vi "FTW-CodeGen-GenerateCode.vi"(0 "State In":T2, 5 "XRef":refnum<vi>, 7 "Terms":T1(array[cluster]), 9 "Diagram":refnum<vi>) -> (4 "State Out":T2, 6 "Reply":string[](array[string]), 8 "Generated Code?":bool)   [LabVIEW 2013, in "FTW-SQLite-Insert.xnode"]
uses:
  FTW-SQLite-Insert.xnode
  FTW-CodeGen-State.ctl
  codegen/FTW-CodeGen.lvlib
panel:
  # "Inputs"
  # "Outputs"
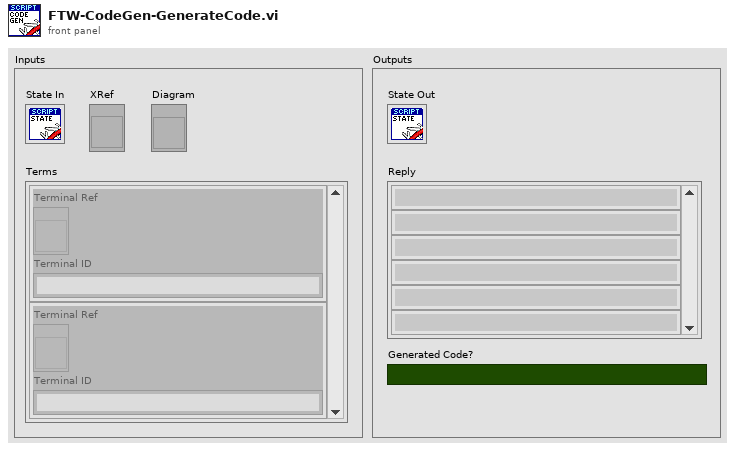
[diagram p1: front panel]
types:
  T1 = cluster{"Terminal Ref":refnum<vi>, "Terminal ID":string}[]
  T2 = typedef "FTW-SQLite-Insert.xnode/FTW-CodeGen-State.ctl" = cluster{"Dummy":string}
  T3 = typedef "LVPositionTypeDef.ctl" = cluster{"Left":i32, "Top":i32}
  T4 = typedef "FTW-Reflection-Types.ctl" = enum16{"Unknown", "Void", "Array", "Cluster", "LVObject", "Boolean", "I8", "I16", "I32", "I64", "U8", "U16", "U32", "U64", "SGL", "DBL", "EXT", "CSG", "CDB", "CXT", "FXP", "EnumU8", "EnumU16", "EnumU32", "EnumU64", "SGLwithUnit", "DBLwithUnit", "EXTwithUnit", "CSGwithUnit", "CDBwithUnit", "CXTwithUnit", "String", "Path", "Picture", "Tag", "LVVariant", "Timestamp", "WaveformI8", "WaveformI16", "WaveformI32", "WaveformI64", "WaveformU8", "WaveformU16", "WaveformU32", "WaveformU64", "WaveformSGL", "WaveformDBL", "WaveformEXT", "WaveformCSG", "WaveformCDB", "WaveformCXT", "WaveformDigital", "WaveformUnknownType", "DigitalData", "DynamicData", "ExternalData", "FileByteStream", "TDMStream", "dotNET", "ActiveX", "VIServerReference", "VIReference", "ApplicationInstance", "Menu", "ConnectionDataSocket", "ConnectionVISA", "ConnectionBluetooth", "ConnectionIrDA", "ConnectionTCP", "ConnectionUDP", "ConnectionHTTPClient", "ConnectionFTP", "Occurrence", "Notifier", "Queue", "Rendezvous", "Semaphore", "RTFIFO", "EventPublisher", "EventRegistration", "EventCallback", "DataValueReference", "GenericClass", "GenericClassTag", "GenericClassDeepCopy", "GenericClassFlattened", "GenericClassTagFlattened", "GenericReferenceType", "WindowsRegistry", "OverloadedDatalogRef", "ReferenceUnknownType"}
  T5 = cluster{"Element Name":string, "Element Type":T4, "Element Value":variant}[]
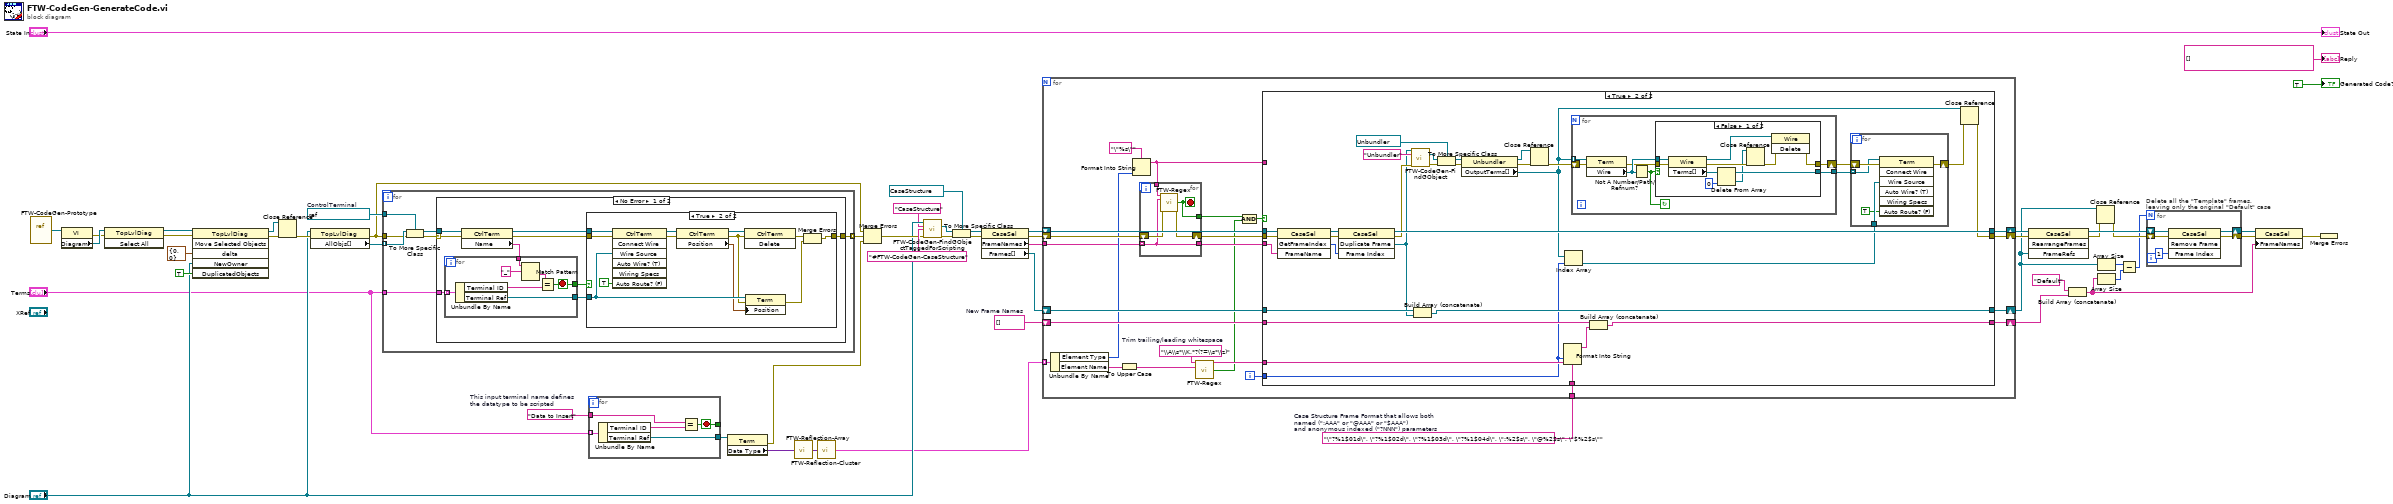
[diagram p0: block diagram]
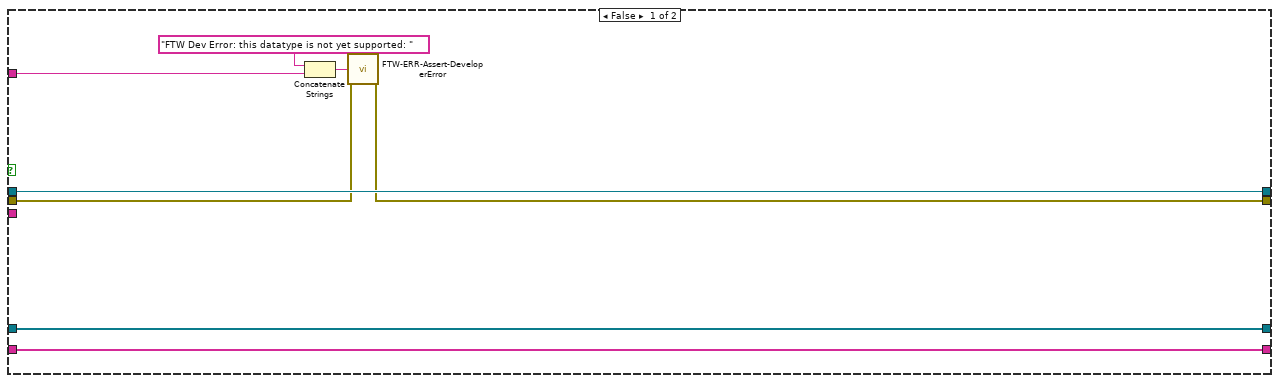
[diagram p2: hidden frame]
diagram:
  w1 = "\"?%1$01d\", \"?%1$02d\", \"?%1$03d\", \"?%1$04d\", \":%2$s\", \"@%2$s\", \"$%2$s\""  # Case Structure Frame Format that allows both named (":AAA" or "@AAA" or "$AAA") and anonymous indexed ("?NNN") parameters
  w19 = string[] []  # New Frame Names
  w31 = "Data to Insert"  # This input terminal name defines the datatype to be scripted
  w49 = refnum<vi> refnum  # ControlTerminal
  n1 = vi-ref "FTW-CodeGen-Prototype.vi"() -> (w42:refnum<vi>)
  n2 = property class="VI"(reference=w42) -> (error out=w41:errorcluster, "Diagram"=w48:refnum<vi>)  [unwired: 1 in, 1 out]
  n3 = invoke class="TopLvlDiag" method="Select All"(reference=w48, error in=w41) -> (reference out=w52:refnum<vi>, error out=w51:errorcluster)  [unwired: 1 in, 1 out]
  n4 = invoke class="TopLvlDiag" method="Move Selected Objects"(reference=w52, error in=w51, "delta"=cluster{"X":i32, "Y":i32} {"X"=0, "Y"=0} ("X/Y Delta"), "NewOwner"="Diagram", "DuplicatedObjects"=TRUE ("Duplicate? (F)")) -> (reference out=w38:refnum<vi>, error out=w40:errorcluster)  [unwired: 1 in, 4 out]
  n5 = Close Reference(reference=w38, error in (no error)=w40) -> (error out=w39:errorcluster)
  n6 = property class="TopLvlDiag"(reference="Diagram", error in=w39) -> (error out=w46:errorcluster, "AllObjs[]"=w50:refnum<vi>[])  [unwired: 1 out]
  n7 = for {
    tunnel: w50 -> [w61] mode=indexing
    tunnel: w46 -> [w60]
    tunnel: w49 -> [w59]
    tunnel: "Terms" -> [w56]
    tunnel: [w55] -> w47 mode=indexing
    n8 = To More Specific Class(target class=w59, reference=w61, error in=w60) -> (specific class reference=w57:refnum<vi>, error out=w58:errorcluster)
    n9 = case shown="No Error" w58 {
      selector: w58 -> [w69 _]
      tunnel: w57 -> [w70 _]
      tunnel: w56 -> [w68 _]
      tunnel: [w63 _] -> w55
      frame No Error {
        n10 = property class="CtrlTerm"(reference=w70, error in=w69) -> (reference out=w65:refnum<vi>, error out=w64:errorcluster, "Name"=w67:string)
        n11 = for {
          tunnel: w68 -> [w90] mode=indexing
          tunnel: w67 -> [w88]
          tunnel: [w89] -> w66
          tunnel: [w84] -> w62
          stop <- w84 stop-if-true
          n12 = Unbundle By Name(w90) -> ("Terminal ID"=w85:string, "Terminal Ref"=w89:refnum<vi>)
          n13 = Match Pattern(string=w88, regular expression="_") -> (after substring=w86:string)  [unwired: 1 in, 3 out]
          n14 = Equal?(x=w86, y=w85) -> (x = y?=w84:bool)
        }
        n15 = case shown="True" w62 {
          tunnel: w66 -> [_ w75]
          tunnel: w65 -> [_ w83]
          tunnel: w64 -> [w71 w82]
          tunnel: [w71 w77] -> w63
          frame False {
          }
          frame True {
            n16 = invoke class="CtrlTerm" method="Connect Wire"(reference=w83, error in=w82, "Wire Source"=w75, "Auto Route? (F)"=TRUE) -> (reference out=w81:refnum<vi>, error out=w79:errorcluster)  [unwired: 3 in, 5 out]
            n17 = property class="CtrlTerm"(reference=w81, error in=w79) -> (reference out=w80:refnum<vi>, error out=w74:errorcluster, "Position"=w72:T3)
            n18 = invoke class="CtrlTerm" method="Delete"(reference=w80, error in=w74) -> (error out=w78:errorcluster)  [unwired: 1 in, 2 out]
            n19 = property class="Term"(reference=w75, error in=w74, "Position"=w72) -> (error out=w73:errorcluster)  [unwired: 1 out]
            n20 = Merge Errors(w78, w73) -> (w77:errorcluster)
          }
        }
      }
      frame Error {
      }
    }
  }
  n21 = for {
    tunnel: "Terms" -> [w95] mode=indexing
    tunnel: [w94] -> w29
    tunnel: [w92] -> _
    tunnel: w31 -> [w91]
    stop <- w92 stop-if-true
    n22 = Unbundle By Name(w95) -> ("Terminal ID"=w93:string, "Terminal Ref"=w94:refnum<vi>)
    n23 = Equal?(x=w91, y=w93) -> (x = y?=w92:bool)
  }
  n24 = property class="Term"(reference=w29) -> (error out=w4:errorcluster, "Data Type"=w3:variant)  [unwired: 1 in, 1 out]
  n25 = call "FTW-Reflection-Array.vi"("Array"=w3) -> ("Default Array Element"=w2:variant)  [unwired: 13 in, 1 out]
  n26 = call "FTW-Reflection-Cluster.vi"("Cluster"=w2) -> ("Cluster Elements"=w28:T5)  [unwired: 14 in]
  n27 = Merge Errors(w46, w47, w4) -> (w36:errorcluster)
  n28 = call "FTW-CodeGen-FindGObjectTaggedForScripting.vi"("GObject to Traverse"="Diagram", "Class Name"="CaseStructure", "Label Prefix to uniquely identify node"="#FTW-CodeGen-CaseStructure" ("Label to uniquely identify node"), "error in"=w36) -> ("GObject"=w35:refnum<vi>, "error out"=w34:errorcluster)  [unwired: 10 in]
  n29 = To More Specific Class(target class=refnum<vi> refnum ("Object"), reference=w35, error in=w34) -> (specific class reference=w27:refnum<vi>, error out=w25:errorcluster)
  n30 = property class="CaseSel"(reference=w27, error in=w25) -> (reference out=w26:refnum<vi>, error out=w24:errorcluster, "FrameNames"=w23:string[], "Frames[]"=w11:refnum<vi>[])
  n31 = for {
    tunnel: w28 -> [w117] mode=indexing
    tunnel: w23 -> [w103]
    shift-right: [w112] -> w16
    shift-left: w26 -> [w119]
    shift-right: [w113] -> w14
    shift-left: w24 -> [w118]
    shift-right: [w111] -> w10
    shift-left: w11 -> [w114]
    shift-right: [w109] -> w17
    shift-left: w19 -> [w110]
    tunnel: w1 -> [w105]
    i -> [w106]
    w99 = "\\A\\s*\\K.*?(?=\\s*\\z)"  # Trim trailing/leading whitespace
    n32 = Unbundle By Name(w117) -> ("Element Type"=w107:T4, "Element Name"=w108:string)
    n33 = To Upper Case(1:w108) -> (0:w101:string)
    n34 = Format Into String(format string="\"%s\"", w107) -> (resulting string=w115:string)  [unwired: 2 in, 1 out]
    n35 = for {
      tunnel: w115 -> [w123]
      shift-right: [w122] -> w104
      shift-left: w118 -> [w124]
      tunnel: w103 -> [w120] mode=indexing
      tunnel: [w121] -> w98
      tunnel: [w120] -> w102
      stop <- w121 stop-if-true
      n36 = call "FTW-Regex.vi"("Regular Expression"=w123, "Input String"=w120, "error in"=w124) -> ("Match Found?"=w121:bool, "error out"=w122:errorcluster)  [unwired: 8 in, 3 out]
    }
    n37 = call "FTW-Regex.vi"("Regular Expression"=w99, "Input String"=w101) -> ("Match"=w100:string, "Match Found?"=w96:bool)  [unwired: 9 in, 3 out]
    n38 = Compound Arithmetic op=AND(w98, w96) -> (w97:bool)
    n39 = case shown="True" w97 {
      tunnel: w104 -> [w126 w159]
      tunnel: w119 -> [w132 w160]
      tunnel: w114 -> [w131 w164]
      tunnel: [w131 w161] -> w111
      tunnel: [w125 w137] -> w113
      tunnel: [w132 w154] -> w112
      tunnel: w110 -> [w130 w163]
      tunnel: [w130 w162] -> w109
      tunnel: w102 -> [_ w155]
      tunnel: w100 -> [_ w136]
      tunnel: w106 -> [_ w135]
      tunnel: w115 -> [w128 _]
      tunnel: w105 -> [_ w134]
      frame False {
        n40 = Concatenate Strings("FTW Dev Error: this datatype is not yet supported: " ("Reason this error should never happen"), w128) -> (w127:string)
        n41 = call "FTW-ERR-Assert-DeveloperError.vi"("Reason this error should never happen"=w127, "error in"=w126) -> ("error out"=w125:errorcluster)  [unwired: 13 in]
      }
      frame True {
        n42 = invoke class="CaseSel" method="GetFrameIndex"(reference=w160, error in=w159, "FrameName"=w155) -> (reference out=w158:refnum<vi>, error out=w157:errorcluster, "GetFrameIndex"=w156:i32)  [unwired: 1 in, 1 out]
        n43 = invoke class="CaseSel" method="Duplicate Frame"(reference=w158, error in=w157, "Frame Index"=w156) -> (reference out=w154:refnum<vi>, error out=w139:errorcluster, "Duplicate Frame"=w138:refnum<vi>)  [unwired: 1 in, 1 out]
        n44 = call "FTW-CodeGen-FindGObject.vi"("GObject to Traverse"=w138, "Class Name"="Unbundler", "error in"=w139) -> ("GObject"=w150:refnum<vi>, "error out"=w151:errorcluster)  [unwired: 11 in]
        n45 = Build Array (concatenate)(w164, w138) -> (w161:refnum<vi>[])
        n46 = To More Specific Class(target class=refnum<vi> refnum ("Object"), reference=w150, error in=w151) -> (specific class reference=w148:refnum<vi>, error out=w147:errorcluster)
        n47 = property class="Unbundler"(reference=w148, error in=w147) -> (reference out=w142:refnum<vi>, error out=w144:errorcluster, "OutputTerms[]"=w141:refnum<vi>[])
        n48 = Close Reference(reference=w142, error in (no error)=w144) -> (error out=w143:errorcluster)
        n49 = Format Into String(format string=w134, w135, w136) -> (resulting string=w153:string)  [unwired: 2 in, 1 out]
        n50 = Index Array(array=w141, index=w135) -> (element=w146:refnum<vi>)
        n51 = for {
          tunnel: w141 -> [w176] mode=indexing
          tunnel: [w173] -> w133
          shift-right: [w170] -> w145
          shift-left: w143 -> [w171]
          stop <- w174 continue-if-true
          n52 = property class="Term"(reference=w176, error in=w171) -> (error out=w172:errorcluster, "Wire"=w175:refnum<vi>)  [unwired: 1 out]
          n53 = Not A Number/Path/Refnum?(number/path/refnum=w175) -> (NaN/Path/Refnum?=w174:bool)
          n54 = case shown="False" w174 {
            tunnel: w175 -> [w186 _]
            tunnel: [w184 _] -> w173
            tunnel: w172 -> [w183 w187]
            tunnel: [w181 w187] -> w170
            frame False {
              n55 = property class="Wire"(reference=w186, error in=w183) -> (reference out=w182:refnum<vi>, error out=w180:errorcluster, "Terms[]"=w185:refnum<vi>[])
              n56 = Delete From Array(array=w185, index=0) -> (deleted portion=w178:refnum<vi>, array with subset deleted=w184:refnum<vi>[])  [unwired: 1 in]
              n57 = Close Reference(reference=w178, error in (no error)=w180) -> (error out=w179:errorcluster)
              n58 = invoke class="Wire" method="Delete"(reference=w182, error in=w179) -> (error out=w181:errorcluster)  [unwired: 1 in, 2 out]
            }
            frame True {
            }
          }
        }
        n59 = Build Array (concatenate)(w163, w153) -> (w162:string[])
        n60 = for {
          tunnel: w146 -> [w169]
          shift-right: [w166] -> w140
          shift-left: w145 -> [w167]
          tunnel: w133 -> [w165] mode=indexing
          n61 = invoke class="Term" method="Connect Wire"(reference=w165, error in=w167, "Wire Source"=w169, "Auto Route? (F)"=TRUE) -> (error out=w166:errorcluster)  [unwired: 3 in, 6 out]
        }
        n62 = Close Reference(reference=w141, error in (no error)=w140) -> (error out=w137:errorcluster)
      }
    }
  }
  n63 = invoke class="CaseSel" method="RearrangeFrames"(reference=w16, error in=w14, "FrameRefs"=w10) -> (reference out=w15:refnum<vi>, error out=w13:errorcluster)  [unwired: 1 in, 2 out]
  n64 = Build Array (concatenate)("Default", w17) -> (w9:string[])
  n65 = Close Reference(reference=w10, error in (no error)=w13) -> (error out=w12:errorcluster)
  n66 = Array Size(array=w10) -> (size(s)=w8:i32)
  n67 = Array Size(array=w9) -> (size(s)=w7:i32)
  n68 = Subtract(x=w8, y=w7) -> (x-y=w6:i32)
  n69 = for "Delete all the \"Template\" frames,\nleaving only the original \"Default\" case" {
    N: w6 -> [_]
    shift-right: [w189] -> w21
    shift-left: w12 -> [w190]
    shift-right: [w191] -> w22
    shift-left: w15 -> [w192]
    n70 = invoke class="CaseSel" method="Remove Frame"(reference=w192, error in=w190, "Frame Index"=u32 1) -> (reference out=w191:refnum<vi>, error out=w189:errorcluster)  [unwired: 1 in, 2 out]
  }
  n71 = property class="CaseSel"(reference=w22, error in=w21, "FrameNames"=w9) -> (error out=w5:errorcluster)  [unwired: 1 out]
  n72 = Merge Errors(w5) -> ()  [unwired: 1 out]
  "State Out" <- "State In"
  "Reply" <- string[] [] ("Reply")
  "Generated Code?" <- TRUE ("Generated Code?")
